vi "Lector_Ingen.vi"() -> ()   [LabVIEW 2017, in "Lib_Maestro_Ingen.lvlib"]
uses:
  Lib_Maestro_Ingen.lvlib
  <vilib>/NI Modbus.llb/MB Ethernet Master Query Read Holding Registers (poly).vi
  <vilib>/NI Modbus.llb/MB Ethernet Master Query Write Multiple Registers (poly).vi
panel:
  in  "Tab Control 3":enum32{"Registro", "Control de variables"}(tab)=enum."Control de variables"
  in  "Tab Control":T1(tab)=enum."Registro de Frecuencia"
  out "Voltaje Fase 3":dbl(graph)=119.45
  out "Voltaje Fase 2":dbl(graph)=135.24
  out "Voltaje Fase 1":dbl(graph)=134.03
  out "Voltaje Promedio":dbl(graph)=233.23
  out "Corriente Promedio":dbl(graph)=53.75
  out "Corriente Fase 1":dbl(graph)=60.84
  out "Corriente Fase 2":dbl(graph)=61.24
  out "Corriente Fase 3":dbl(graph)=39.16
  out "Potencia Fase 3":dbl(graph)=76.8
  out "Potencia Fase 2":dbl(graph)=84.51
  out "Potencia Fase 1":dbl(graph)=83.64
  out "Potencia Promedio":dbl(graph)=81.65
  out "Factor de Potencia Fase 3":dbl(graph)=90.57
  out "Factor de Potencia Fase 2":dbl(graph)=90.84
  out "Factor de Potencia Fase 1":dbl(graph)=90.36
  out "Factor de Potencia Promedio":dbl(graph)=90.59
  out "Frecuencia":dbl(graph)=60.18
  in  "Tab Control 2":T2(tab)
  in  "CONTROL TEMPERATURA":cluster{"SET POINT":dbl, "INC T":dbl}={"SET POINT"=50.0, "INC T"=1.0}
  out "TEMPERATURA ACTUAL":dbl(slide)=31.0 scale=0.0..100.0
  out "Tempratura":cluster{"Dato":dbl, "SET POINT":dbl}(graph)
  out "Presion":cluster{"Dato":dbl, "SET POINT":dbl}(graph)
  in  "CONTROL DE PRESIÓN":cluster{"SET POINT":dbl, "INC P":dbl}={"SET POINT"=50.0, "INC P"=1.0}
  out "PRESIÓN ACTUAL":dbl(knob)=50.0 scale=0.0..200.0
  out "Humedad":cluster{"Dato":dbl, "SET POINT":dbl}(graph)
  in  "CONTROL DE HUMEDAD":cluster{"SET POINT":dbl, "INC %":dbl}={"SET POINT"=50.0, "INC %"=1.0}
  out "HUMEDAD ACTUAL":dbl(knob)=50.0 scale=0.0..100.0
  out "Volumen":cluster{"Dato":dbl, "SET POINT":dbl}(graph)
  in  "CONTROL DE LLENADO":cluster{"SET POINT":dbl, "INC  L":dbl}={"SET POINT"=25.0, "INC  L"=1.0}
  out "VOLUMEN ACTUAL":dbl(slide)=25.0 scale=0.0..100.0
  out "error out":errorcluster
  in  "Stop":bool
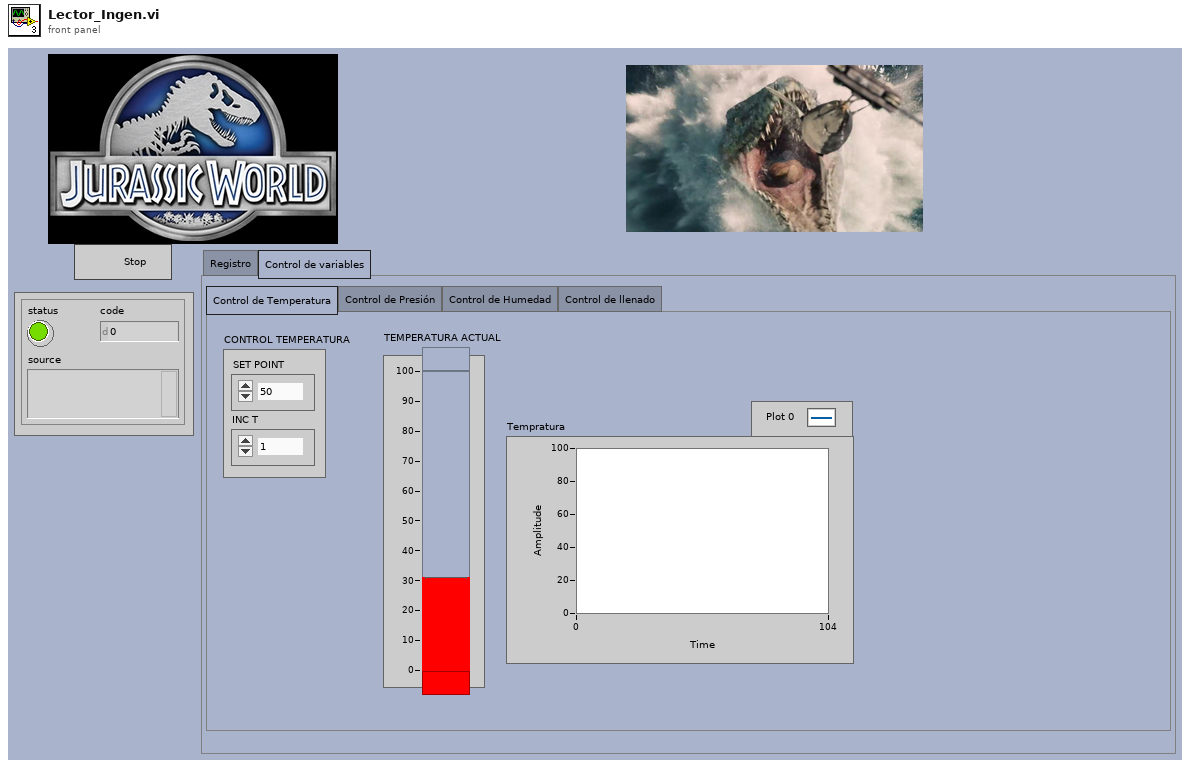
[diagram p1: front panel]
types:
  T1 = enum32{"Registro de Tensión", "Registro de Corriente", "Registro de Potencia", "Registro de Factor de Potencia", "Registro de Frecuencia"}
  T2 = enum32{"Control de Temperatura", "Control de Presión", "Control de Humedad", "Control de llenado"}
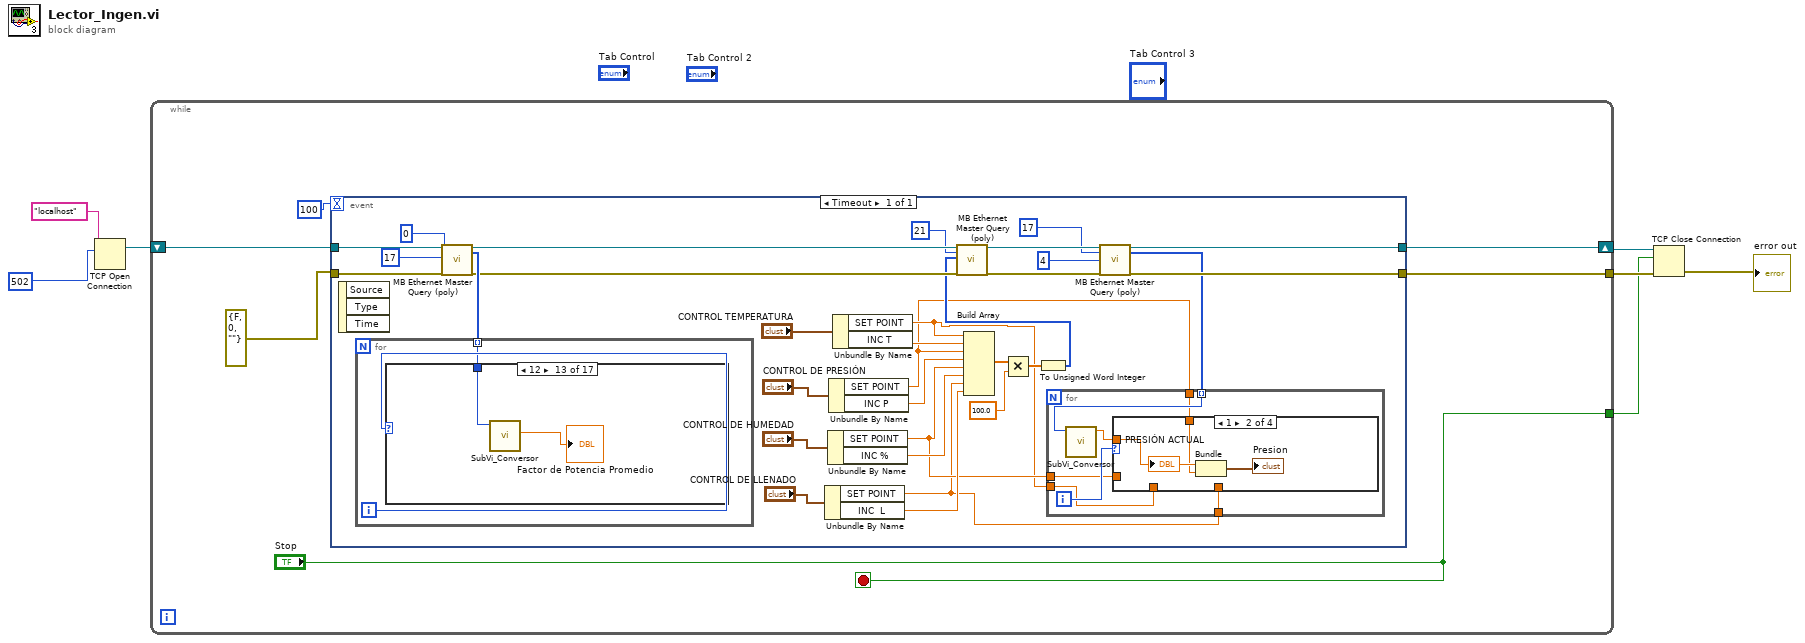
[diagram p0: block diagram]
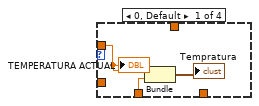
[diagram p2: hidden frame]
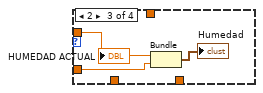
[diagram p3: hidden frame]
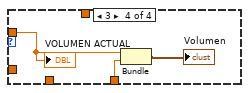
[diagram p4: hidden frame]
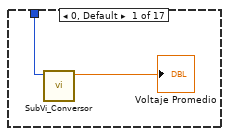
[diagram p5: hidden frame]
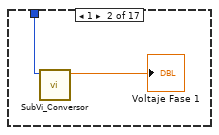
[diagram p6: hidden frame]
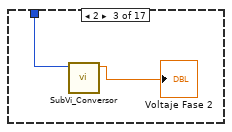
[diagram p7: hidden frame]
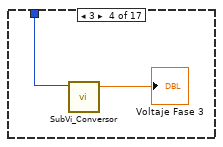
[diagram p8: hidden frame]
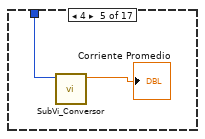
[diagram p9: hidden frame]
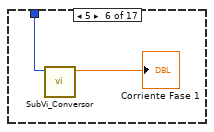
[diagram p10: hidden frame]
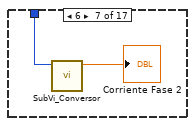
[diagram p11: hidden frame]
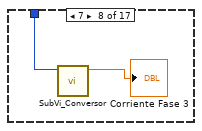
[diagram p12: hidden frame]
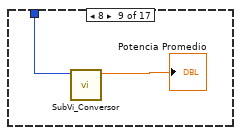
[diagram p13: hidden frame]
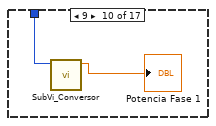
[diagram p14: hidden frame]
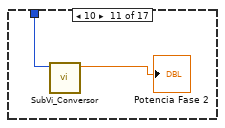
[diagram p15: hidden frame]
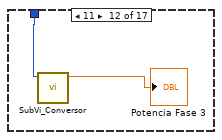
[diagram p16: hidden frame]
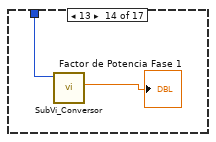
[diagram p17: hidden frame]
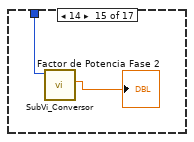
[diagram p18: hidden frame]
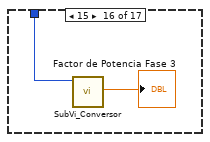
[diagram p19: hidden frame]
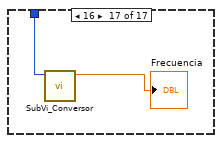
[diagram p20: hidden frame]
diagram:
  n1 = TCP Open Connection(address="localhost", remote port or service name=u16 502) -> (connection ID=w5:refnum<k5>)  [unwired: 3 in, 1 out]
  n2 = while {
    tunnel: [w11] -> w3
    shift-right: [w12] -> w4
    shift-left: w5 -> [w10]
    tunnel: ["Stop"] -> w2
    stop <- "Stop" stop-if-true
    n3 = event shown="[0] Timeout" {
      selector: _ -> [_]
      dyn-events: _ -> [_]
      timeout: 100 -> [_]
      tunnel: w10 -> [w44]
      tunnel: errorcluster {"status"=FALSE, "code"=0, "source"=""} ("error out") -> [w43]
      tunnel: [w20] -> w12
      tunnel: [w19] -> w11
      event Timeout {
        n4 = event-data() -> ()  [unwired: 1 in, 3 out]
        n5 = call-poly <vilib>:"MB Ethernet Master Query (poly).vi"("TCP Connection Refnum in"=w44, "Starting Address"=u16 0, "Quantity"=u16 17, "error in"=w43) -> ("TCP Connection Refnum (dup)"=w28:refnum<k5>, "Holding Registers"=w40:u16[], "error out"=w27:errorcluster)  [unwired: 12 in, 1 out]
        n6 = for {
          tunnel: w40 -> [w64] mode=indexing
          i -> [w65]
          n7 = case shown="12" w65 {
            tunnel: w64 -> [w67 w68 w71 w72 w75 w77 w79 w81 w83 w85 w87 w88 w90 w93 w95 w96 w98]
            frame 0, Default {
              n8 = call "SubVi_Conversor.vi"("Entrada_U16"=w67) -> ("Dato"=→"Voltaje Promedio":dbl)  [unwired: 9 in, 1 out]
            }
            frame 1 {
              n9 = call "SubVi_Conversor.vi"("Entrada_U16"=w68) -> ("Dato"=→"Voltaje Fase 1":dbl)  [unwired: 9 in, 1 out]
            }
            frame 2 {
              n10 = call "SubVi_Conversor.vi"("Entrada_U16"=w71) -> ("Dato"=→"Voltaje Fase 2":dbl)  [unwired: 9 in, 1 out]
            }
            frame 3 {
              n11 = call "SubVi_Conversor.vi"("Entrada_U16"=w72) -> ("Dato"=→"Voltaje Fase 3":dbl)  [unwired: 9 in, 1 out]
            }
            frame 4 {
              n12 = call "SubVi_Conversor.vi"("Entrada_U16"=w75) -> ("Dato"=→"Corriente Promedio":dbl)  [unwired: 9 in, 1 out]
            }
            frame 5 {
              n13 = call "SubVi_Conversor.vi"("Entrada_U16"=w77) -> ("Dato"=→"Corriente Fase 1":dbl)  [unwired: 9 in, 1 out]
            }
            frame 6 {
              n14 = call "SubVi_Conversor.vi"("Entrada_U16"=w79) -> ("Dato"=→"Corriente Fase 2":dbl)  [unwired: 9 in, 1 out]
            }
            frame 7 {
              n15 = call "SubVi_Conversor.vi"("Entrada_U16"=w81) -> ("Dato"=→"Corriente Fase 3":dbl)  [unwired: 9 in, 1 out]
            }
            frame 8 {
              n16 = call "SubVi_Conversor.vi"("Entrada_U16"=w83) -> ("Dato"=→"Potencia Promedio":dbl)  [unwired: 9 in, 1 out]
            }
            frame 9 {
              n17 = call "SubVi_Conversor.vi"("Entrada_U16"=w85) -> ("Dato"=→"Potencia Fase 1":dbl)  [unwired: 9 in, 1 out]
            }
            frame 10 {
              n18 = call "SubVi_Conversor.vi"("Entrada_U16"=w87) -> ("Dato"=→"Potencia Fase 2":dbl)  [unwired: 9 in, 1 out]
            }
            frame 11 {
              n19 = call "SubVi_Conversor.vi"("Entrada_U16"=w88) -> ("Dato"=→"Potencia Fase 3":dbl)  [unwired: 9 in, 1 out]
            }
            frame 12 {
              n20 = call "SubVi_Conversor.vi"("Entrada_U16"=w90) -> ("Factor_de_potencia"=→"Factor de Potencia Promedio":dbl)  [unwired: 9 in, 1 out]
            }
            frame 13 {
              n21 = call "SubVi_Conversor.vi"("Entrada_U16"=w93) -> ("Factor_de_potencia"=→"Factor de Potencia Fase 1":dbl)  [unwired: 9 in, 1 out]
            }
            frame 14 {
              n22 = call "SubVi_Conversor.vi"("Entrada_U16"=w95) -> ("Factor_de_potencia"=→"Factor de Potencia Fase 2":dbl)  [unwired: 9 in, 1 out]
            }
            frame 15 {
              n23 = call "SubVi_Conversor.vi"("Entrada_U16"=w96) -> ("Factor_de_potencia"=→"Factor de Potencia Fase 3":dbl)  [unwired: 9 in, 1 out]
            }
            frame 16 {
              n24 = call "SubVi_Conversor.vi"("Entrada_U16"=w98) -> ("Dato"=→"Frecuencia":dbl)  [unwired: 9 in, 1 out]
            }
          }
        }
        n25 = Unbundle By Name("CONTROL DE LLENADO") -> ("SET POINT"=w16:dbl, "INC  L"=w32:dbl)
        n26 = Unbundle By Name("CONTROL DE HUMEDAD") -> ("SET POINT"=w17:dbl, "INC %"=w33:dbl)
        n27 = Unbundle By Name("CONTROL DE PRESIÓN") -> ("SET POINT"=w14:dbl, "INC P"=w34:dbl)
        n28 = Unbundle By Name("CONTROL TEMPERATURA") -> ("SET POINT"=w15:dbl, "INC T"=w35:dbl)
        n29 = Build Array(w15, w35, w14, w34, w17, w33, w16, w32) -> (w31:dbl[])
        n30 = Multiply(x=w31, y=100.0) -> (x*y=w29:dbl[])
        n31 = To Unsigned Word Integer(number=w29) -> (unsigned 16bit integer=w25:u16[])
        n32 = call-poly <vilib>:"MB Ethernet Master Query (poly).vi"("TCP Connection Refnum in"=w28, "Starting Address"=u16 21, "Registers"=w25, "error in"=w27) -> ("TCP Connection Refnum (dup)"=w24:refnum<k5>, "error out"=w23:errorcluster)  [unwired: 13 in, 1 out]
        n33 = call-poly <vilib>:"MB Ethernet Master Query (poly).vi"("TCP Connection Refnum in"=w24, "Starting Address"=u16 17, "Quantity"=u16 4, "error in"=w23) -> ("TCP Connection Refnum (dup)"=w20:refnum<k5>, "Holding Registers"=w18:u16[], "error out"=w19:errorcluster)  [unwired: 12 in, 1 out]
        n34 = for {
          tunnel: w18 -> [w51] mode=indexing
          tunnel: w17 -> [w48]
          tunnel: w16 -> [w47]
          tunnel: w15 -> [w46]
          tunnel: w14 -> [w45]
          i -> [w50]
          n35 = call "SubVi_Conversor.vi"("Entrada_U16"=w51) -> ("Dato"=w49:dbl)  [unwired: 9 in, 1 out]
          n36 = case shown="1" w50 {
            tunnel: w49 -> [w53 w56 w60 w62]
            tunnel: w48 -> [_ _ w58 _]
            tunnel: w47 -> [_ _ _ w61]
            tunnel: w46 -> [w52 _ _ _]
            tunnel: w45 -> [_ w55 _ _]
            frame 0, Default {
              n37 = Bundle("Dato"=w53, "SET POINT"=w52) -> (→"Tempratura":cluster{"Dato":dbl, "SET POINT":dbl})  [unwired: 1 in]
              "TEMPERATURA ACTUAL" <- w53
            }
            frame 1 {
              n38 = Bundle("Dato"=w56, "SET POINT"=w55) -> (→"Presion":cluster{"Dato":dbl, "SET POINT":dbl})  [unwired: 1 in]
              "PRESIÓN ACTUAL" <- w56
            }
            frame 2 {
              n39 = Bundle("Dato"=w60, "SET POINT"=w58) -> (→"Humedad":cluster{"Dato":dbl, "SET POINT":dbl})  [unwired: 1 in]
              "HUMEDAD ACTUAL" <- w60
            }
            frame 3 {
              n40 = Bundle("Dato"=w62, "SET POINT"=w61) -> (→"Volumen":cluster{"Dato":dbl, "SET POINT":dbl})  [unwired: 1 in]
              "VOLUMEN ACTUAL" <- w62
            }
          }
        }
      }
    }
  }
  n41 = TCP Close Connection(connection ID=w4, abort (F)=w2, error in (no error)=w3) -> (error out=→"error out":errorcluster)  [unwired: 1 out]
